vi "EOL CAN_Check Calibration status.vi"(8 "error in (no error)":errorcluster, 9 "Glass?":bool, 10 "Read Session in":refnum<k21>, 11 "Write Session in":refnum<k21>) -> (0 "error out":errorcluster, 1 "Calibrated":bool, 2 "Response Good?":bool, 3 "TxRx Data":string[][](array[string]))   [LabVIEW 2014]
uses:
  <vilib>/xnet/xnet.llb/XNET Frame CAN.ctl
  <vilib>/xnet/xnet.llb/XNET Frame Type CAN.ctl
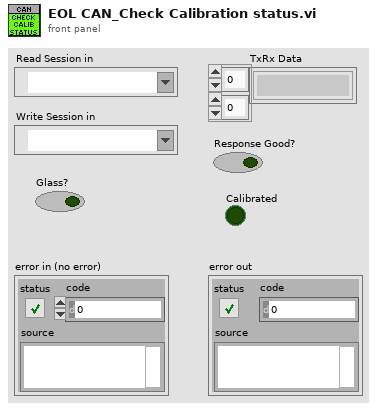
[diagram p1: front panel]
types:
  T1 = typedef "XNET Frame CAN.ctl" = cluster{"timestamp":timestamp, "payload":u8[], "identifier":u32, "type":T2, "extended?":bool, "echo?":bool}
  T2 = typedef "XNET Frame Type CAN.ctl" = u8
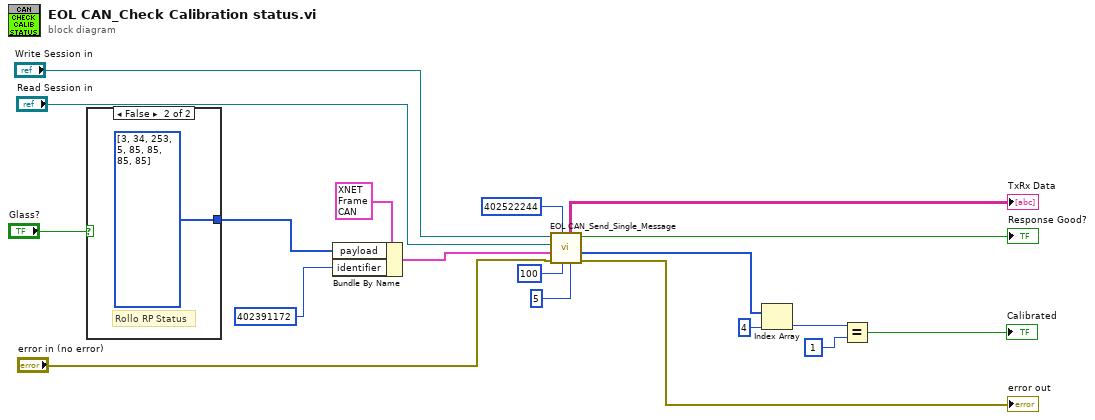
[diagram p0: block diagram]
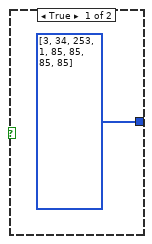
[diagram p2: hidden frame]
diagram:
  n1 = case shown="False" "Glass?" {
    tunnel: [u8[] [3, 34, 253, 1, 85, 85, 85, 85] ("payload") u8[] [3, 34, 253, 5, 85, 85, 85, 85] ("payload")] -> w18
    frame True {
    }
    frame False {
      # "Rollo RP Status"
    }
  }
  n2 = Bundle By Name(cluster=T1 {"timestamp"=timestamp(0 s since 1904-01-01), "payload"=[2, 39, 3, 85, 85, 85, 85, 85], "identifier"=402391172, "type"=0, "extended?"=TRUE, "echo?"=FALSE} ("Tx CAN frame"), "payload"=w18, "identifier"=u32 402391172) -> (w17:T1)
  n3 = call "EOL CAN_Send_Single_Message.vi"("Retries"=5, "Msg Wait Time"=u32 100, "Rx Arbitration Id"=u32 402522244, "Error in"="error in (no error)", "Tx CAN frame"=w17, "Read Session in"="Read Session in", "Write Session in"="Write Session in") -> ("Error out"=→"error out":errorcluster, "Rx Message"=w5:u8[], "Response Good?"=→"Response Good?":bool, "TxRx Data"=→"TxRx Data":string[][])  [unwired: 1 out]
  n4 = Index Array(array=w5, index=4) -> (element=w3:u8)
  n5 = Equal?(x=w3, y=u8 1) -> (x = y?=→"Calibrated":bool)
